vi "UpdateNowTips.vi"(10 "NewVersionOnWeb":string, 11 "LangSet":u32) -> (3 "UpdateNow":bool)   [LabVIEW 2015]
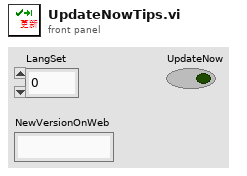
[diagram p1: front panel]
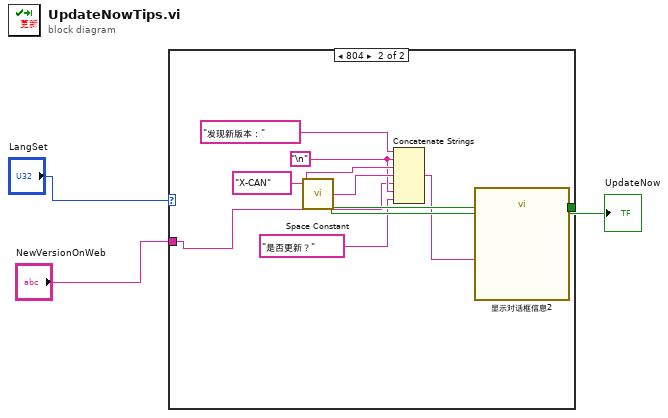
[diagram p0: block diagram]
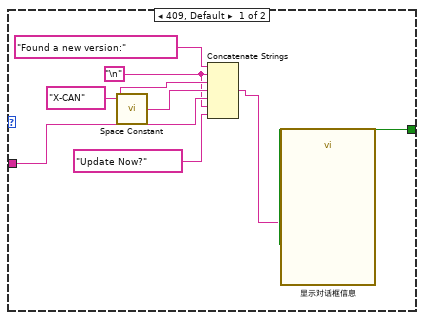
[diagram p2: hidden frame]
diagram:
  n1 = case shown="804" "LangSet" {
    tunnel: [w11 w19] -> w1
    tunnel: "NewVersionOnWeb" -> [w7 w13]
    frame 409, Default {
      w6 = "\n"
      n2 = call <vilib>:"Space Constant.vi"() -> ("String"=w8:string)
      n3 = Concatenate Strings("Found a new version:", w6, "X-CAN", w8, w7, w6, "Update Now?") -> (w4:string)
      n4 = call "显示对话框信息"("Message"=w4) -> ("UpdateNow"=w11:bool)  [unwired: 9 in, 1 out]
    }
    frame 804 {
      w15 = "\n"
      n5 = call <vilib>:"Space Constant.vi"() -> ("String"=w16:string)
      n6 = Concatenate Strings("发现新版本：", w15, "X-CAN", w16, w13, w15, "是否更新？") -> (w12:string)
      n7 = call "显示对话框信息2"("Message"=w12) -> ("立即更新"=w19:bool)  [unwired: 9 in, 1 out]
    }
  }
  "UpdateNow" <- w1
